vi "Force By Wire.vi"(8 "error in (no error)":errorcluster, 11 "Carya Config in":refnum<class "Carya Config (By Reference).lvclass">) -> (0 "error out":errorcluster, 2 "Carya Config out":refnum<class "Carya Config.lvclass">, 3 "Carya Config out":refnum<class "Carya Config (By Reference).lvclass">)   [LabVIEW 2013, in "Carya Config (By Reference).lvclass"]
doc: "Copyright 2018, Carya Automatisering, Wiebe Walstra."
uses:
  Carya Config (By Reference).lvclass
  Carya Config.lvclass
  CConfig Buffer Type/CConfig Buffer Type.lvclass
  Carya Config (By Reference).lvclass/Carya Config (By Reference).ctl
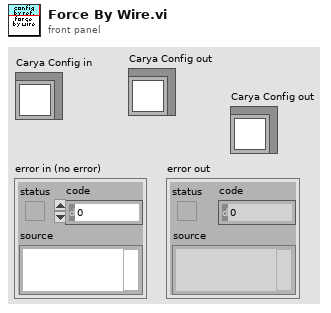
[diagram p1: front panel]
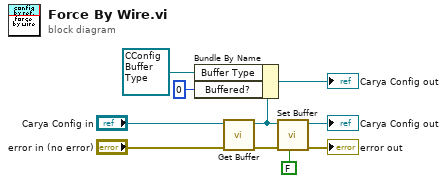
[diagram p0: block diagram]
diagram:
  n1 = call-dynamic "Get Buffer.vi"("error in (no error)"="error in (no error)", "Carya Config in"="Carya Config in") -> ("error out"=w8:errorcluster, "Config"=w3:refnum<class "Carya Config (By Reference).lvclass">)  [unwired: 8 in]
  n2 = Bundle By Name(cluster=w3, "Buffer Type"=refnum<class "CConfig Buffer Type.lvclass"> refnum, "Buffered?"=0) -> (→"Carya Config out":refnum<class "Carya Config (By Reference).lvclass">)
  n3 = call-dynamic "Set Buffer.vi"("Set? [T]"=FALSE, "error in (no error)"=w8, "Carya Config"=w3) -> ("error out"=→"error out":errorcluster, "Carya Config out"=→"Carya Config out":refnum<class "Carya Config (By Reference).lvclass">)  [unwired: 7 in]
